vi "DAQOutputControlVCA.vi"() -> ()   [LabVIEW 2015]
panel:
  out "Control Voltage Display":dbl
  in  "stop":bool
  out "Gauge":dbl(knob) scale=0.0..10.0
  in  "Manually Set Voltage":dbl
  # "EE2073\nGROUP 1"
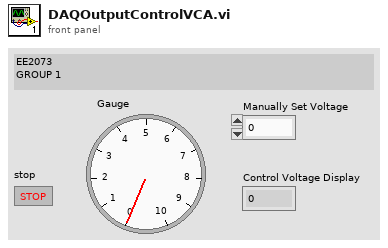
[diagram p1: front panel]
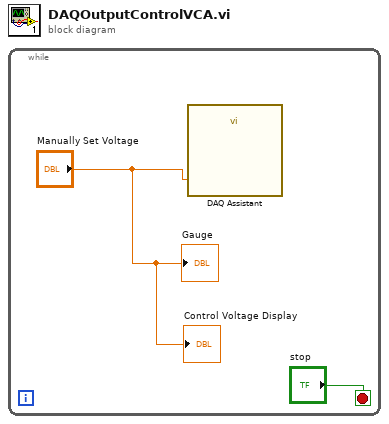
[diagram p0: block diagram]
diagram:
  n1 = while {
    stop <- "stop" stop-if-true
    n2 = call "DAQ Assistant"("data"="Manually Set Voltage") -> ()  [unwired: 17 in, 2 out]
    "Gauge" <- "Manually Set Voltage"
    "Control Voltage Display" <- "Manually Set Voltage"
  }
